vi "Byte Buffer Mapping.vi"() -> ()   [LabVIEW 2016]
uses:
  Source/Library/Typedefs/Typedefs.Data Types.ctl
  Source/Library/Byte Buffer/Byte Buffer.lvclass/Byte Buffer.ctl
  Source/Library/Byte Buffer/Byte Buffer.Mapping.Create (Channel Pointer).vi
  Source/Library/SubVIs/Sizeof.Array.vi
  Source/Library/Memory Management/Memory Management.MoveDblBlock.Write (Double).vi
  Source/Library/Byte Buffer/Byte Buffer.Mapping.Write Typed Array.vi
  Source/Library/SubVIs/Buffer.Double.vi
  Source/Library/Byte Buffer/Byte Buffer.Mapping.Read Typed Array.vi
  Source/Library/Memory Management/Memory Management.MoveDblBlock.Read (Double).vi
  Source/Library/SubVIs/Sizeof.Scalar.vi
  Source/Library/Byte Buffer/Byte Buffer.Write.vi
  Source/Library/Byte Buffer/Byte Buffer.Write (1D Boolean).vi
  Source/Library/Type Conversion/Type Conversion.From Double.Subset.vi
  Source/Library/Type Conversion/Type Conversion.From Double.Subset (1D Boolean).vi
  Source/Library/Byte Buffer/Byte Buffer.Write (1D SGL).vi
  Source/Library/Type Conversion/Type Conversion.From Double.Subset (1D SGL).vi
  Source/Library/Byte Buffer/Byte Buffer.Write (1D DBL).vi
  Source/Library/Byte Buffer/Byte Buffer.Write (1D I8).vi
  Source/Library/Type Conversion/Type Conversion.From Double.Subset (1D I8).vi
  Source/Library/Byte Buffer/Byte Buffer.Write (1D I16).vi
  Source/Library/Type Conversion/Type Conversion.From Double.Subset (1D I16).vi
  Source/Library/Byte Buffer/Byte Buffer.Write (1D I32).vi
  Source/Library/Type Conversion/Type Conversion.From Double.Subset (1D I32).vi
  Source/Library/Byte Buffer/Byte Buffer.Write (1D I64).vi
  Source/Library/Type Conversion/Type Conversion.From Double.Subset (1D I64).vi
  Source/Library/Byte Buffer/Byte Buffer.Write (1D U8).vi
  Source/Library/Type Conversion/Type Conversion.From Double.Subset (1D U8).vi
  Source/Library/Byte Buffer/Byte Buffer.Write (1D U16).vi
  Source/Library/Type Conversion/Type Conversion.From Double.Subset (1D U16).vi
  Source/Library/Byte Buffer/Byte Buffer.Write (1D U32).vi
  Source/Library/Type Conversion/Type Conversion.From Double.Subset (1D U32).vi
  Source/Library/Byte Buffer/Byte Buffer.Write (1D U64).vi
  Source/Library/Type Conversion/Type Conversion.From Double.Subset (1D U64).vi
  Source/Library/Byte Buffer/Byte Buffer.Read.vi
  Source/Library/Byte Buffer/Byte Buffer.Read (1D Boolean).vi
  Source/Library/Type Conversion/Type Conversion.To Double.Subset.vi
  Source/Library/Type Conversion/Type Conversion.To Double.Subset (1D Boolean).vi
  Source/Library/Byte Buffer/Byte Buffer.Read (1D SGL).vi
  Source/Library/Type Conversion/Type Conversion.To Double.Subset (1D SGL).vi
  Source/Library/Byte Buffer/Byte Buffer.Read (1D DBL).vi
  Source/Library/Byte Buffer/Byte Buffer.Read (1D I8).vi
  Source/Library/Type Conversion/Type Conversion.To Double.Subset (1D I8).vi
  Source/Library/Byte Buffer/Byte Buffer.Read (1D I16).vi
  Source/Library/Type Conversion/Type Conversion.To Double.Subset (1D I16).vi
  Source/Library/Byte Buffer/Byte Buffer.Read (1D I32).vi
  Source/Library/Type Conversion/Type Conversion.To Double.Subset (1D I32).vi
  Source/Library/Byte Buffer/Byte Buffer.Read (1D I64).vi
  Source/Library/Type Conversion/Type Conversion.To Double.Subset (1D I64).vi
  Source/Library/Byte Buffer/Byte Buffer.Read (1D U8).vi
  Source/Library/Type Conversion/Type Conversion.To Double.Subset (1D U8).vi
  Source/Library/Byte Buffer/Byte Buffer.Read (1D U16).vi
  Source/Library/Type Conversion/Type Conversion.To Double.Subset (1D U16).vi
  Source/Library/Byte Buffer/Byte Buffer.Read (1D U32).vi
  Source/Library/Type Conversion/Type Conversion.To Double.Subset (1D U32).vi
  Source/Library/Byte Buffer/Byte Buffer.Read (1D U64).vi
  Source/Library/Type Conversion/Type Conversion.To Double.Subset (1D U64).vi
  Source/Library/Type Conversion/Type Conversion.From Double.vi
  Source/Library/Type Conversion/Type Conversion.From Double (1D Boolean).vi
  Source/Library/Type Conversion/Type Conversion.From Double (1D SGL).vi
  Source/Library/Type Conversion/Type Conversion.From Double (1D I8).vi
  Source/Library/Type Conversion/Type Conversion.From Double (1D I16).vi
  Source/Library/Type Conversion/Type Conversion.From Double (1D I32).vi
  Source/Library/Type Conversion/Type Conversion.From Double (1D I64).vi
  Source/Library/Type Conversion/Type Conversion.From Double (1D U8).vi
  Source/Library/Type Conversion/Type Conversion.From Double (1D U16).vi
  Source/Library/Type Conversion/Type Conversion.From Double (1D U32).vi
  Source/Library/Type Conversion/Type Conversion.From Double (1D U64).vi
  Source/Library/Type Conversion/Type Conversion.To Double.vi
  Source/Library/Type Conversion/Type Conversion.To Double (1D Boolean).vi
  Source/Library/Type Conversion/Type Conversion.To Double (1D SGL).vi
  Source/Library/Type Conversion/Type Conversion.To Double (1D I8).vi
  Source/Library/Type Conversion/Type Conversion.To Double (1D I16).vi
  Source/Library/Type Conversion/Type Conversion.To Double (1D I32).vi
  Source/Library/Type Conversion/Type Conversion.To Double (1D I64).vi
  Source/Library/Type Conversion/Type Conversion.To Double (1D U8).vi
  Source/Library/Type Conversion/Type Conversion.To Double (1D U16).vi
  Source/Library/Type Conversion/Type Conversion.To Double (1D U32).vi
  Source/Library/Type Conversion/Type Conversion.To Double (1D U64).vi
  Source/Library/Memory Management/Memory Management.Handle Return.vi
  Source/Library/Byte Buffer/Byte Buffer.lvclass
  Source/Library/VeriStand Data.lvlib
panel:
  out "Required Buffer Size":i32 format="%.0f bytes"
  out "error out":errorcluster
  in  "Data to Write":dbl[](array[numeric]) format="%#.3f"
  in  "stop":bool
  out "buffer":string
  in  "Data Types":T1[](array[typedef])=[enum."I16", enum."Boolean", enum."I32", enum."Single", enum."Double", enum."Double", enum."U32", enum."U64"]
  in  "Byte Order":T2(ring)=enum."little-endian"
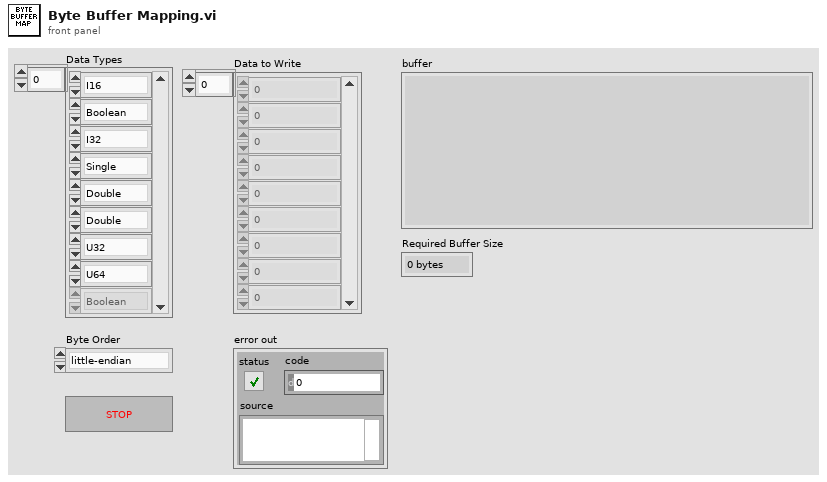
[diagram p1: front panel]
types:
  T1 = typedef "VeriStand Data.lvlib/Typedefs.Data Types.ctl" = enum16{"Boolean", "Single", "Double", "I8", "I16", "I32", "I64", "U8", "U16", "U32", "U64"}
  T2 = enum16{"big-endian, network order", "native, host order", "little-endian"}
  T3 = typedef "VeriStand Data.lvlib/Byte Buffer.lvclass/Byte Buffer.Mapping.ctl" = cluster{"pointer":u64, "count":i32, "buffer offset":i32, "data type":T1}
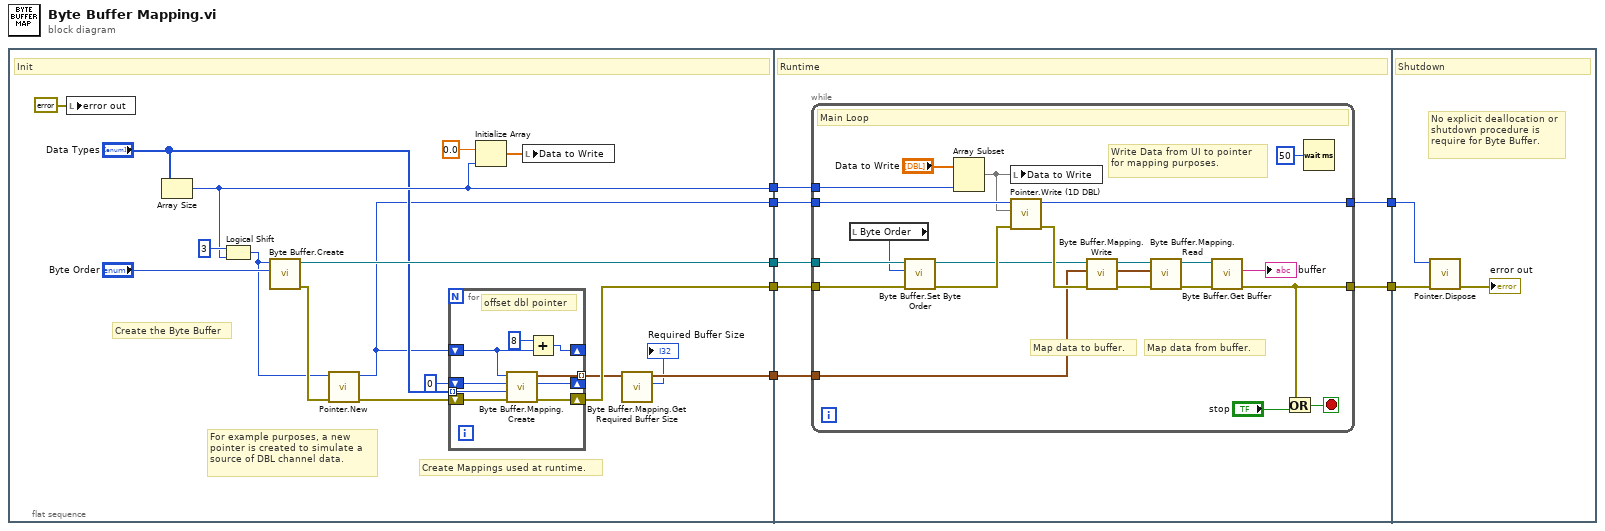
[diagram p0: block diagram]
diagram:
  n1 = flat-sequence {
    tunnel: [w21] -> w7
    tunnel: [w18] -> w6
    tunnel: [w9] -> w5
    tunnel: [w16] -> w4
    tunnel: [w14] -> w3
    tunnel: w7 -> [w40]
    tunnel: w6 -> [w39]
    tunnel: w5 -> [w38]
    tunnel: w4 -> [w37]
    tunnel: w3 -> [w36]
    tunnel: [w35] -> w2
    tunnel: [w34] -> w1
    tunnel: w2 -> [w64]
    tunnel: w1 -> [w65]
    frame #0 {
      # "Create Mappings used at runtime."
      # "Create the Byte Buffer"
      # "For example purposes, a new pointer is created to simulate a source of DBL channel data."
      # "Init"
      n2 = local write "error out"(errorcluster {"status"=FALSE, "code"=0, "source"=""} ("error out")) -> ()
      n3 = Array Size(array="Data Types") -> (size(s)=w16:i32)
      n4 = Logical Shift(y=i16 3, x=w16) -> (x << y=w19:i32)
      n5 = call "Byte Buffer.Create.vi"("byte order (big-endian)"="Byte Order", "size"=w19) -> ("error out"=w22:errorcluster, "Byte Buffer"=w21:refnum<class "Byte Buffer.lvclass">)  [unwired: 8 in]
      n6 = call "Pointer.New.vi"("error in (no error)"=w22, "size in bytes"=w19) -> ("error out"=w20:errorcluster, "pointer"=w14:u64)  [unwired: 8 in]
      n7 = for {
        tunnel: [w33] -> w10 mode=indexing
        tunnel: "Data Types" -> [w30] mode=indexing
        shift-right: [w31] -> w18
        shift-left: w20 -> [w32]
        shift-right: [w28] -> _
        shift-left: w14 -> [w29]
        shift-right: [w26] -> _
        shift-left: 0 ("buffer offset") -> [w25]
        # "offset dbl pointer"
        n8 = call-poly "Byte Buffer.Mapping.Create.vi"("error in (no error)"=w32, "data type"=w30, "buffer offset"=w25, "Channel Pointer"=w29) -> ("error out"=w31:errorcluster, "new buffer offset"=w26:i32, "mapping"=w33:T3)  [unwired: 5 in]
        n9 = Add(x=u64 8, y=w29) -> (x+y=w28:u64)
      }
      n10 = Initialize Array(0.0 ("element"), w16) -> (w13:dbl[])
      n11 = local write "Data to Write"(w13) -> ()
      n12 = call "Byte Buffer.Mapping.Get Required Buffer Size.vi"("mappings"=w10) -> ("required buffer size"=→"Required Buffer Size":i32, "mappings dup"=w9:T3[])  [unwired: 9 in]
    }
    frame #1 {
      # "Runtime"
      n13 = while {
        tunnel: w40 -> [w47]
        tunnel: w39 -> [w46]
        tunnel: w38 -> [w41]
        tunnel: w37 -> [w55]
        tunnel: w36 -> [w53]
        tunnel: [w48] -> w35
        tunnel: [w42] -> w34
        stop <- w50 stop-if-true
        # "Write Data from UI to pointer for mapping purposes."
        # "Map data from buffer."
        # "Map data to buffer."
        # "Main Loop"
        n14 = local read "Byte Order"() -> (w43:T2)
        n15 = call "Byte Buffer.Set Byte Order.vi"("error in (no error)"=w46, "byte order"=w43, "Byte Buffer in"=w47) -> ("error out"=w45:errorcluster, "Byte Buffer out"=w44:refnum<class "Byte Buffer.lvclass">)  [unwired: 7 in]
        n16 = Array Subset(array="Data to Write", length=w55) -> (w52:dbl[])  [unwired: 1 in]
        n17 = local write "Data to Write"(w52) -> ()
        n18 = call "Pointer.Write (1D DBL).vi"("error in (no error)"=w45, "values"=w52, "pointer in"=w53) -> ("error out"=w62:errorcluster, "pointer out"=w42:u64)  [unwired: 6 in, 1 out]
        n19 = call "Byte Buffer.Mapping.Write.vi"("error in (no error)"=w62, "mappings"=w41, "Byte Buffer in"=w44) -> ("error out"=w59:errorcluster, "mappings dup"=w61:T3[], "Byte Buffer out"=w60:refnum<class "Byte Buffer.lvclass">)  [unwired: 6 in]
        n20 = call "Byte Buffer.Mapping.Read.vi"("error in (no error)"=w59, "mappings"=w61, "Byte Buffer in"=w60) -> ("error out"=w57:errorcluster, "Byte Buffer out"=w58:refnum<class "Byte Buffer.lvclass">)  [unwired: 6 in, 1 out]
        n21 = call "Byte Buffer.Get Buffer.vi"("error in (no error)"=w57, "Byte Buffer in"=w58) -> ("error out"=w48:errorcluster, "buffer"=→"buffer":string)  [unwired: 7 in, 1 out]
        n22 = Or(x=w48, y="stop") -> (x .or. y?=w50:bool)
        n23 = Wait (ms)(milliseconds to wait=u32 50) -> ()  [unwired: 1 out]
      }
    }
    frame #2 {
      # "No explicit deallocation or shutdown procedure is require for Byte Buffer."
      # "Shutdown"
      n24 = call "Pointer.Dispose.vi"("error in (no error)"=w64, "pointer"=w65) -> ("error out"=→"error out":errorcluster)  [unwired: 8 in, 1 out]
    }
  }
